vi "透明的vi背景.vi"() -> ()   [LabVIEW 2016]
uses:
  user32.dll
panel:
  out "前面板背景色":u32=16448250 format="%.0x"
  out "错误输出":errorcluster
  in  "错误输入（无错误）":errorcluster
  in  "停止":bool
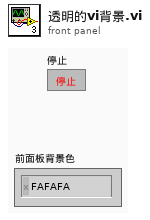
[diagram p1: front panel]
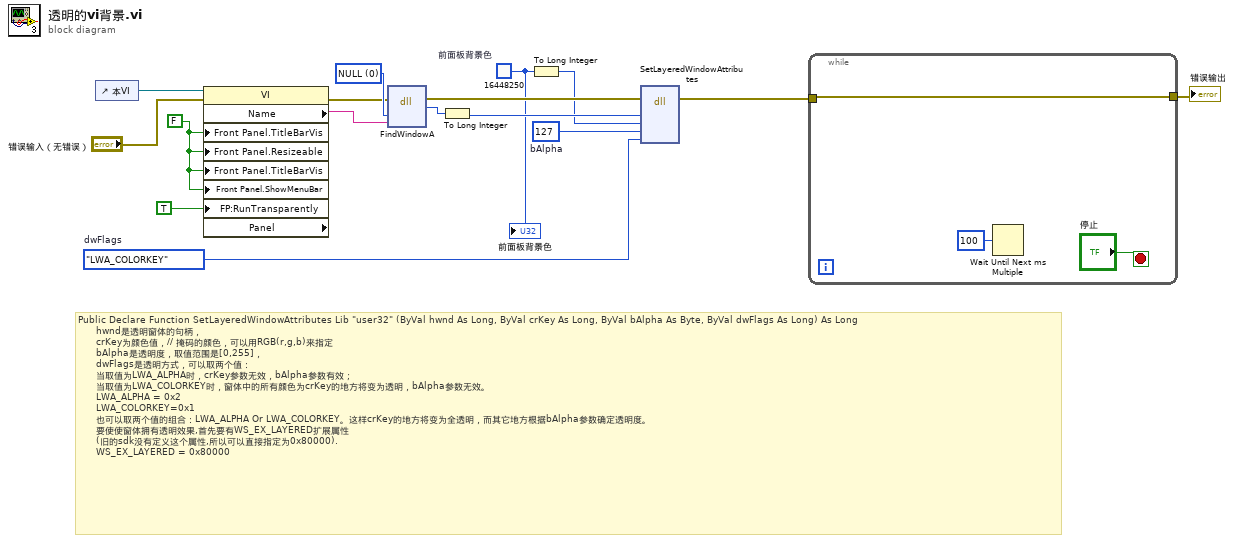
[diagram p0: block diagram]
diagram:
  w2 = FALSE
  w4 = u32 16448250  # 前面板背景色
  w12 = u8 127  # bAlpha
  w10 = enum16{"NONE", "LWA_COLORKEY", "LWA_ALPHA"}."LWA_COLORKEY"  # dwFlags
  w16 = 0 items=["NULL"]
  # "Public Declare Function SetLayeredWindowAttributes Lib \"user32\" (ByVal hwnd As Long, ByVal crKey As Long, ByVal bAlpha As Byte, ByVal dwFlags As Long) As Long\n　　hwnd是透明窗体的句柄，\n　　crKey为颜色值，// 掩码的颜色，可以用RGB(r,g,b)来指定\n　　bAlpha是透明度，取值范围是[0,255]，\n　　dwFlags是透明方式，可以取两个值：\n　　当取值为LWA_ALPHA时，crKey参数无效，bAlpha参数有效；\n　　当取值为LWA_COLORKEY时，窗体中的所有颜色为crKey的地方将变为透明，bAlpha参数无效。\n　　LWA_ALPHA = 0x2\n　　LWA_COLORKEY=0x1\n　　也可以取两个值的组合：LWA_ALPHA Or LWA_COLORKEY。这样crKey的地方将变为全透明，而其它地方根据bAlpha参数确定透明度。\n　　要使使窗体拥有透明效果,首先要有WS_EX_LAYERED扩展属性\n　　(旧的sdk没有定义这个属性,所以可以直接指定为0x80000). \n　　WS_EX_LAYERED = 0x80000"
  n1 = control-ref of="本VI"() -> (w5:refnum<vi>)
  n2 = property class="VI" props=["Name", "Front Panel.TitleBarVis", "Front Panel.Resizeable", "Front Panel.TitleBarVis", "Front Panel.ShowMenuBar", "FP:RunTransparently", "Panel"](reference=w5, error in="错误输入（无错误）", "Front Panel.TitleBarVis"=w2, "Front Panel.Resizeable"=w2, "Front Panel.TitleBarVis"=w2, "Front Panel.ShowMenuBar"=w2, "FP:RunTransparently"=TRUE) -> (error out=w13:errorcluster, "Name"=w15:string)  [unwired: 2 out]
  n3 = dll-call lib="user32.dll" fn="FindWindowA" label="FindWindow"(error in=w13, "lpszClassName"=w16, "lpszWindowName"=w15) -> (error out=w9:errorcluster, "hWnd"=w14:u32)  [unwired: 4 in, 1 out]
  n4 = To Long Integer(number=w14) -> (32bit integer=w11:i32)
  n5 = To Long Integer(number=w4) -> (32bit integer=w3:i32)
  n6 = dll-call lib="user32.dll" fn="SetLayeredWindowAttributes" label="SetLayeredWindowAttributs"(error in=w9, "handle"=w11, "crkey"=w3, "bAlpha"=w12, "dwFlags"=w10) -> (error out=w7:errorcluster)  [unwired: 4 in, 4 out]
  n7 = while {
    tunnel: w7 -> [w17]
    tunnel: [w17] -> w6
    stop <- "停止" stop-if-true
    n8 = Wait Until Next ms Multiple(millisecond multiple=u32 100 ("毫秒倍数")) -> ()  [unwired: 1 out]
  }
  "错误输出" <- w6
  "前面板背景色" <- w4
